vi "Finish.vi"   [LabVIEW 2015]
doc: "This VI is called just before exiting. It is expected to close I/O refnum, save collected data, etc."
uses:
  <vilib>/Rock Robotics/WPI/Utilities/WPI_GetSetVariantRefNum.vi
types:
  T1 = typedef "WPI_MotorControlDeviceRef.ctl" = cluster{"DeviceStatus":errorcluster, "Type":T2, "PWM":cluster{"PWM Channel":T3, "DeadBand":T4}, "CAN":cluster{"Device Number":u8, "Control Mode":T5, "Semaphore":T6, "Max Vout":dbl, "TalonSRX Control Mode":T7}, "Invert":bool}
  T2 = typedef "WPI_MotorControlType.ctl" = enum16{"PWM", "CAN", "CANTalonSRX"}
  T3 = typedef "FPGA_DIOPWMChannel.ctl" = enum8{"PWM 0", "PWM 1", "PWM 2", "PWM 3", "PWM 4", "PWM 5", "PWM 6", "PWM 7", "PWM 8", "PWM 9", "PWM MXP 0", "PWM MXP 1", "PWM MXP 2", "PWM MXP 3", "PWM MXP 4", "PWM MXP 5", "PWM MXP 6", "PWM MXP 7", "PWM MXP 8", "PWM MXP 9", "Invalid"}
  T4 = typedef "WPI_PWMDeadband.ctl" = cluster{"Name":string, "maxPositivePwm":i32, "minPositivePwm":i32, "centerPwm":i32, "maxNegativePwm":i32, "minNegativePwm":i32, "angularRange":u16}
  T5 = typedef "WPI_CANJaguar_ControlMode.ctl" = enum8{"Percent VBus", "Current", "Speed", "Position", "Voltage"}
  T6 = typedef "Semaphore RefNum" = refnum<k1>
  T7 = typedef "WPI_CANTalonSRX_APIControlMode.ctl" = enum8{"Percent VBus", "Speed", "Position", "Slave", "Unchanged / Invalid", "Voltage Compensation", "Current", "Motion Profile"}
  T8 = typedef "WPI_GyroDevRef.ctl" = cluster{"DevStatus":errorcluster, "Analog Channel":T9, "Offset":dbl, "Gain (VoltsPerDegree/Second)":dbl, "Gyro Type":enum16{"Analog", "XRS450"}, "Handle":i32, "SPI Bus":T10, "Device Found":bool, "Sample Rate":dbl, "Calibrate On Open":bool}
  T9 = typedef "FPGA_AIChannel.ctl" = enum8{"AI 0", "AI 1", "AI 2", "AI 3", "AI MXP 0", "AI MXP 1", "AI MXP 2", "AI MXP 3", "Invalid"}
  T10 = typedef "spi_bus.ctl" = enum16{"SPI On-Board, CS0", "SPI On-Board, CS1", "SPI On-Board, CS2", "SPI On-Board, CS3", "SPI MXP", "Invalid"}
  T11 = typedef "WPI_JoystickDevRef.ctl" = cluster{"Device":T12}
  T12 = typedef "WPI_JoystickDeviceEnum.ctl" = enum16{"USB 0", "USB 1", "USB 2", "USB 3", "USB 4", "USB 5"}
  T13 = typedef "WPI_RobotDriveDevRef.ctl" = cluster{"DevStatus":errorcluster, "Motors[]":T1[], "Square Inputs":bool, "Max Output":dbl}
  T14 = typedef "WPI_SolenoidDevRef.ctl" = cluster{"DevStatus":errorcluster, "Pneumatics Control Module":u8, "Forward Solenoid Channel":T15, "Reverse Solenoid Channel":T15}
  T15 = typedef "WPI_SolenoidChannel.ctl" = enum8{"Solenoid 0", "Solenoid 1", "Solenoid 2", "Solenoid 3", "Solenoid 4", "Solenoid 5", "Solenoid 6", "Solenoid 7", "Invalid"}
  T16 = typedef "WPI_DigitalInputDevRef.ctl" = cluster{"DevStatus":errorcluster, "DIO Channel":T17}
  T17 = typedef "FPGA_DIOChannel.ctl" = enum8{"DIO 0", "DIO 1", "DIO 2", "DIO 3", "DIO 4", "DIO 5", "DIO 6", "DIO 7", "DIO 8", "DIO 9", "DIO MXP 0", "DIO MXP 1", "DIO MXP 2", "DIO MXP 3", "DIO MXP 4", "DIO MXP 5", "DIO MXP 6", "DIO MXP 7", "DIO MXP 8", "DIO MXP 9", "DIO MXP 10", "DIO MXP 11", "DIO MXP 12", "DIO MXP 13", "DIO MXP 14", "DIO MXP 15", "Invalid"}
  T18 = typedef "WPI_AccelerometerDevRef.ctl" = cluster{"DevStatus":errorcluster, "Scaling":T19, "Analog Channels":T20, "I2C Bus":T21, "SPI Bus":T10, "Accel Range":T22, "ADXL Axes":T23, "Handle":i32, "Device Address":u8, "Accel Type":enum16{"Analog", "ADXL345 I2C", "ADXL345 SPI", "Internal", "ADXL362 SPI"}}
  T19 = typedef "WPI_AccelerometerScaling.ctl" = cluster{"Gain (VoltsPerG)":dbl, "Center Voltage":dbl}
  T20 = typedef "WPI_AccelerometerAnalogChannels.ctl" = cluster{"X-Axis":T9, "Y-Axis":T9, "Z-Axis":T9}
  T21 = typedef "i2c_bus.ctl" = enum16{"I2C On-Board", "I2C MXP", "Invalid"}
  T22 = typedef "ADXL345 Range.ctl" = u8
  T23 = typedef "WPI_AccelerometerADXL345 Axes.ctl" = cluster{"X-Axis":bool, "Y-Axis":bool, "Z-Axis":bool}
  T24 = typedef "WPI_ServoDeviceRef.ctl" = cluster{"DeviceStatus":errorcluster, "PWM Channel":T3, "DeadBand":T4}
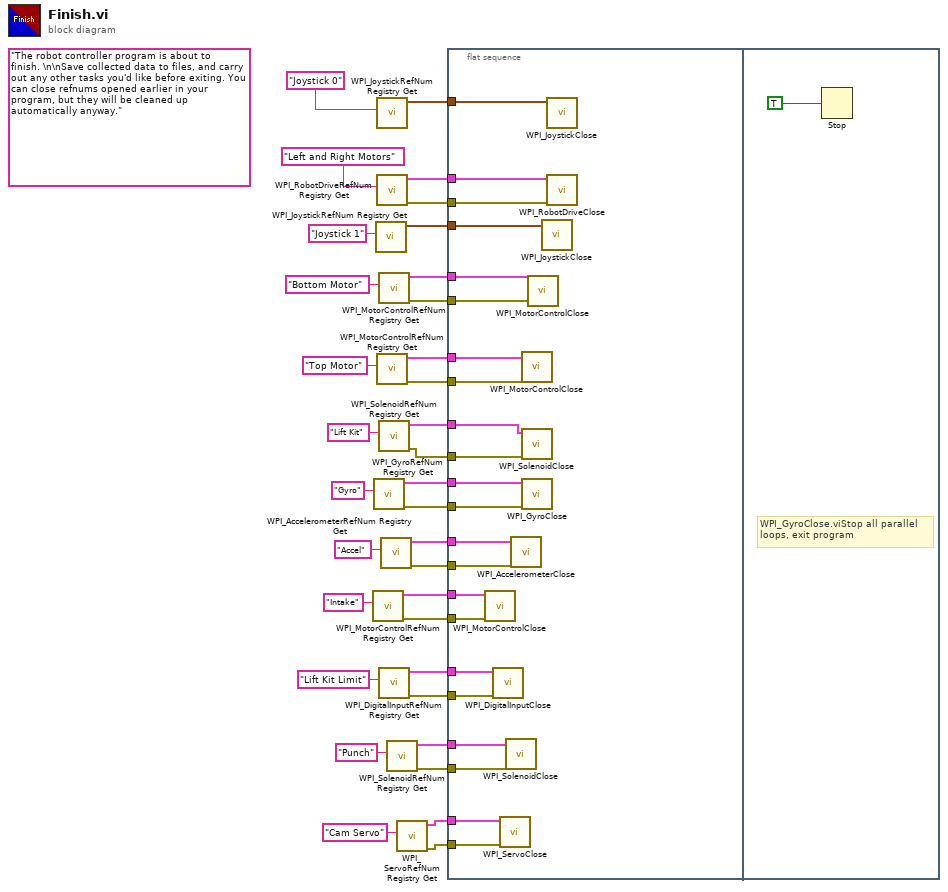
[diagram p0: block diagram]
diagram:
  (unwired) "The robot controller program is about to finish. \n\nSave collected data to files, and carry out any other tasks you'd like before exiting. You can close refnums opened earlier in your program, but they will be cleaned up automatically anyway."
  n1 = call <vilib>:"WPI_MotorControlRefNum Registry Get.vi"("refnum name"="Intake") -> ("error out"=w17:errorcluster, "MotorControlDevRef"=w16:T1)  [unwired: 9 in]
  n2 = call <vilib>:"WPI_GyroRefNum Registry Get.vi"("refnum name"="Gyro") -> ("error out"=w21:errorcluster, "GyroDevRef"=w22:T8)  [unwired: 9 in]
  n3 = call <vilib>:"WPI_JoystickRefNum Registry Get.vi"("refnum name"="Joystick 1") -> ("JoystickDevRef"=w11:T11)  [unwired: 1 in, 9 out]
  n4 = call <vilib>:"WPI_JoystickRefNum Registry Get.vi"("refnum name"="Joystick 0") -> ("JoystickDevRef"=w31:T11)  [unwired: 1 in, 9 out]
  n5 = call <vilib>:"WPI_RobotDriveRefNum Registry Get.vi"("refnum name"="Left and Right Motors") -> ("error out"=w19:errorcluster, "RobotDriveDevRef"=w32:T13)  [unwired: 1 in, 8 out]
  n6 = call <vilib>:"WPI_MotorControlRefNum Registry Get.vi"("refnum name"="Top Motor") -> ("error out"=w20:errorcluster, "MotorControlDevRef"=w29:T1)  [unwired: 9 in]
  n7 = call <vilib>:"WPI_MotorControlRefNum Registry Get.vi"("refnum name"="Bottom Motor") -> ("error out"=w18:errorcluster, "MotorControlDevRef"=w30:T1)  [unwired: 9 in]
  n8 = call <vilib>:"WPI_SolenoidRefNum Registry Get.vi"("refnum name"="Lift Kit") -> ("error out"=w25:errorcluster, "SolenoidDevRef"=w26:T14)  [unwired: 9 in]
  n9 = call <vilib>:"WPI_DigitalInputRefNum Registry Get.vi"("refnum name"="Lift Kit Limit") -> ("error out"=w12:errorcluster, "DigitalInputDevRef"=w14:T16)  [unwired: 9 in]
  n10 = call <vilib>:"WPI_AccelerometerRefNum Registry Get.vi"("refnum name"="Accel") -> ("error out"=w8:errorcluster, "AccelerometerDevRef"=w9:T18)  [unwired: 9 in]
  n11 = call <vilib>:"WPI_SolenoidRefNum Registry Get.vi"("refnum name"="Punch") -> ("error out"=w5:errorcluster, "SolenoidDevRef"=w6:T14)  [unwired: 9 in]
  n12 = call <vilib>:"WPI_ServoRefNum Registry Get.vi"("refnum name"="Cam Servo") -> ("error out"=w2:errorcluster, "ServoDeviceRef"=w3:T24)  [unwired: 9 in]
  n13 = flat-sequence {
    tunnel: w32 -> [w56]
    tunnel: w31 -> [w55]
    tunnel: w30 -> [w54]
    tunnel: w29 -> [w53]
    tunnel: w26 -> [w52]
    tunnel: w25 -> [w51]
    tunnel: w22 -> [w50]
    tunnel: w21 -> [w49]
    tunnel: w20 -> [w48]
    tunnel: w19 -> [w47]
    tunnel: w18 -> [w46]
    tunnel: w17 -> [w45]
    tunnel: w16 -> [w44]
    tunnel: w14 -> [w43]
    tunnel: w12 -> [w42]
    tunnel: w11 -> [w41]
    tunnel: w9 -> [w40]
    tunnel: w8 -> [w39]
    tunnel: w6 -> [w38]
    tunnel: w5 -> [w37]
    tunnel: w3 -> [w36]
    tunnel: w2 -> [w35]
    frame #0 {
      n14 = call <vilib>:"WPI_MotorControlClose.vi"("error in (no error)"=w45, "MotorControlDevRef"=w44) -> ()  [unwired: 9 in, 1 out]
      n15 = call <vilib>:"WPI_DigitalInputClose.vi"("error in (no error)"=w42, "DigitalInputDevRef"=w43) -> ()  [unwired: 9 in, 1 out]
      n16 = call <vilib>:"WPI_ServoClose.vi"("error in (no error)"=w35, "ServoDeviceRef"=w36) -> ()  [unwired: 9 in, 1 out]
      n17 = call <vilib>:"WPI_SolenoidClose.vi"("error in (no error)"=w37, "SolenoidDevRef"=w38) -> ()  [unwired: 9 in, 1 out]
      n18 = call <vilib>:"WPI_AccelerometerClose.vi"("error in"=w39, "AccelerometerDevRef"=w40) -> ()  [unwired: 9 in, 1 out]
      n19 = call <vilib>:"WPI_MotorControlClose.vi"("error in (no error)"=w48, "MotorControlDevRef"=w53) -> ()  [unwired: 9 in, 1 out]
      n20 = call <vilib>:"WPI_SolenoidClose.vi"("error in (no error)"=w51, "SolenoidDevRef"=w52) -> ()  [unwired: 9 in, 1 out]
      n21 = call <vilib>:"WPI_GyroClose.vi"("error in"=w49, "GyroDevRef"=w50) -> ()  [unwired: 9 in, 1 out]
      n22 = call <vilib>:"WPI_MotorControlClose.vi"("error in (no error)"=w46, "MotorControlDevRef"=w54) -> ()  [unwired: 9 in, 1 out]
      n23 = call <vilib>:"WPI_JoystickClose.vi"("JoystickDevRef"=w41) -> ()  [unwired: 11 out]
      n24 = call <vilib>:"WPI_JoystickClose.vi"("JoystickDevRef"=w55) -> ()  [unwired: 11 out]
      n25 = call <vilib>:"WPI_RobotDriveClose.vi"("error in (no error)"=w47, "RobotDriveDevRef"=w56) -> ()  [unwired: 10 out]
    }
    frame #1 {
      # "WPI_GyroClose.viStop all parallel\nloops, exit program"
      n26 = Stop(stop? (T)=TRUE ("Quit")) -> ()
    }
  }
